vi "Modify Dependency Package Version in Package BuildSpec Example.vi"() -> ()   [LabVIEW 2018]
uses:
  Package Build Specification API (2018)/NIPKG BuildSpec API.lvlib
panel:
  in  "Package build spec name":string
  in  "LabVIEW project filepath":path
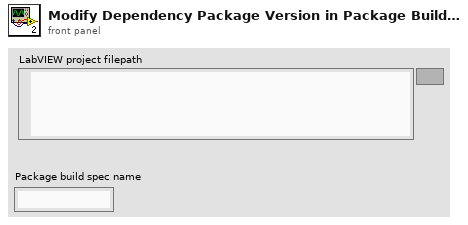
[diagram p1: front panel]
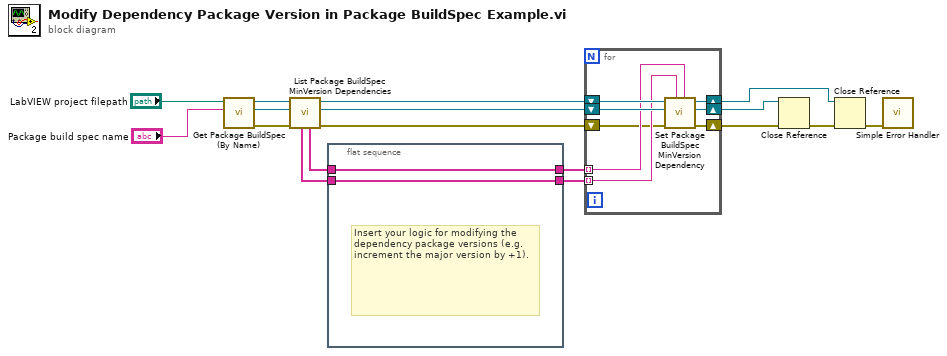
[diagram p0: block diagram]
diagram:
  n1 = call "Get Package BuildSpec (By Name).vi"("package build spec name"="Package build spec name", "LabVIEW project filepath"="LabVIEW project filepath") -> ("error out"=w7:errorcluster, "package build spec ref out"=w12:refnum<vi>, "project ref out"=w13:refnum<vi>)  [unwired: 7 in]
  n2 = call "List Package BuildSpec MinVersion Dependencies.vi"("error in (no error)"=w7, "package buildspec ref in"=w12, "project ref in"=w13) -> ("error out"=w6:errorcluster, "package buildspec ref out"=w10:refnum<vi>, "project ref out"=w11:refnum<vi>, "dependency package names"=w4:string[], "dependency package min versions"=w2:string[])  [unwired: 4 in]
  n3 = flat-sequence {
    tunnel: w4 -> [w19]
    tunnel: [w19] -> w3
    tunnel: w2 -> [w18]
    tunnel: [w18] -> w1
    frame #0 {
      # "Insert your logic for modifying the dependency package versions (e.g. increment the major version by +1)."
    }
  }
  n4 = for {
    tunnel: w3 -> [w25] mode=indexing
    shift-right: [w24] -> w9
    shift-left: w11 -> [w27]
    shift-right: [w23] -> w8
    shift-left: w10 -> [w26]
    tunnel: w1 -> [w22] mode=indexing
    shift-right: [w20] -> w5
    shift-left: w6 -> [w21]
    n5 = call "Set Package BuildSpec MinVersion Dependency.vi"("dependency package name"=w25, "version"=w22, "error in (no error)"=w21, "package buildspec ref in"=w26, "project ref in"=w27) -> ("error out"=w20:errorcluster, "package buildspec ref out"=w23:refnum<vi>, "project ref out"=w24:refnum<vi>)  [unwired: 3 in, 1 out]
  }
  n6 = Close Reference(reference=w8, error in (no error)=w5) -> (error out=w17:errorcluster)
  n7 = Close Reference(reference=w9, error in (no error)=w17) -> (error out=w16:errorcluster)
  n8 = call <vilib>:"Simple Error Handler.vi"("error in (no error)"=w16) -> ()  [unwired: 4 in, 5 out]
